vi "fetch_position_feedback.vi"(8 "error in (no error)":errorcluster, 11 "ScanHeadDL090202 in":refnum<class "ScanHeadDL090202.lvclass">) -> (0 "error out":errorcluster, 3 "ScanHeadDL090202 out":refnum<class "ScanHeadDL090202.lvclass">)   [LabVIEW 2010, in "ScanHeadDL090202.lvclass"]
uses:
  ScanHeadDL090202.lvclass
  common/enumerations/functional_global_action_enum.ctl
  Trajectory/TrajectoryDL091126GenericVoxel/TrajectoryDL091126GenericVoxel/TrajectoryDL091126GenericVoxel.lvclass
  common/classes/ErrorController/ErrorController/ErrorController.lvclass
  internal_trigger_enum.ctl
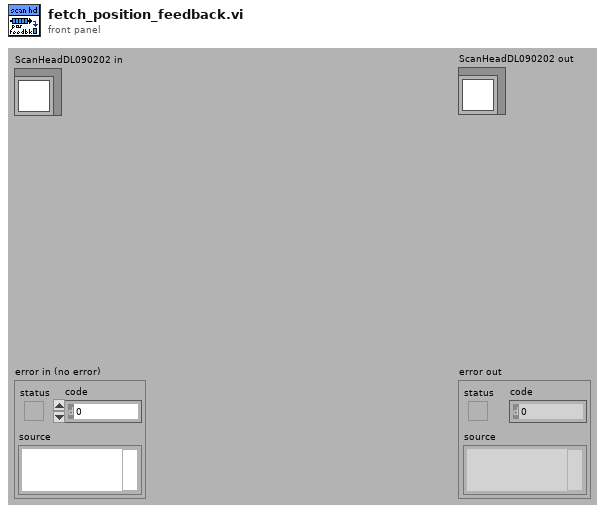
[diagram p1: front panel]
types:
  T1 = typedef "functional_global_action_enum.ctl" = enum16{"get", "set", "reset"}
  T2 = typedef "ScanHeadDL090202.lvclass/internal_trigger_enum.ctl" = enum16{"NULL", "initialise", "terminate", "start scanning", "stop scanning", "scale", "rotate", "tilt", "translate", "update modifiers", "fetch trajectory", "set run mode", "initialise scanners", "terminate scanners", "generate trajectory", "prepare writing", "write", "calculate scanner delays", "fetch position feedback"}
  T3 = typedef "pixel_raw_data_array.ctl" = dbl[][]
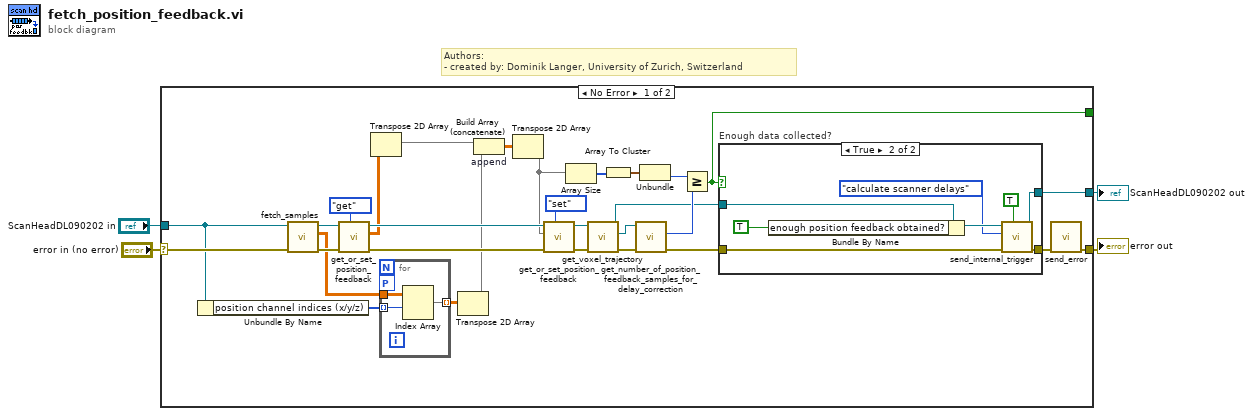
[diagram p0: block diagram]
diagram:
  # "Authors: \n- created by: Dominik Langer, University of Zurich, Switzerland"
  n1 = case shown="No Error" "error in (no error)" {
    selector: "error in (no error)" -> [w9 w49]
    tunnel: [w11 w49] -> w3
    tunnel: [w30 w48] -> w1
    tunnel: "ScanHeadDL090202 in" -> [w8 w48]
    tunnel: [w27 _] -> _
    frame No Error {
      n2 = Unbundle By Name(w8) -> ("position channel indices (x/y/z)"=w25:i32[])
      n3 = call-dynamic "fetch_samples.vi"("error in (no error)"=w9, "GenericToplevelComponent in"=w8) -> ("error out"=w7:errorcluster, "channels raw data block"=w5:T3, "GenericToplevelComponent out"=w6:refnum<class "ScanHeadDL090202.lvclass">)  [unwired: 6 in, 1 out]
      n4 = call-dynamic "get_or_set_position_feedback.vi"("action"=functional_global_action_enum."get", "error in (no error)"=w7, "ScanHeadDL090202 in"=w6) -> ("error out"=w34:errorcluster, "position feedback data out"=w17:T3, "ScanHeadDL090202 out"=w33:refnum<class "ScanHeadDL090202.lvclass">)  [unwired: 6 in]
      n5 = Transpose 2D Array(2D array=w17) -> (transposed array=w16:T3)
      n6 = for {
        tunnel: w25 -> [w36] mode=indexing
        tunnel: w5 -> [w37]
        workers-P: _ -> [_]
        tunnel: [w35] -> w13 mode=indexing
        n7 = Index Array(array=w37, index (row)=w36) -> (element=w35:dbl[])  [unwired: 1 in]
      }
      n8 = Transpose 2D Array(2D array=w13) -> (transposed array=w14:dbl[][])
      n9 = Build Array (concatenate) "append"(w16, w14) -> (w15:T3)
      n10 = Transpose 2D Array(2D array=w15) -> (transposed array=w12:T3)
      n11 = call-dynamic "get_or_set_position_feedback.vi"("action"=functional_global_action_enum."set", "error in (no error)"=w34, "position feedback data in"=w12, "ScanHeadDL090202 in"=w33) -> ("error out"=w24:errorcluster, "ScanHeadDL090202 out"=w20:refnum<class "ScanHeadDL090202.lvclass">)  [unwired: 5 in, 1 out]
      n12 = Array Size(array=w12) -> (size(s)=w29:i32[])
      n13 = call-dynamic "get_voxel_trajectory.vi"("error in (no error)"=w24, "ScanHeadDL090202 in"=w20) -> ("error out"=w22:errorcluster, "trajectory"=w21:refnum<class "TrajectoryDL091126GenericVoxel.lvclass">, "ScanHeadDL090202 out"=w18:refnum<class "ScanHeadDL090202.lvclass">)  [unwired: 7 in]
      n14 = Array To Cluster(array=w29) -> (cluster=w28:cluster{"[0]":i32, "[1]":i32})
      n15 = call-dynamic "get_number_of_position_feedback_samples_for_delay_correction.vi"("error in (no error)"=w22, "TrajectoryDL091126GenericVoxel in"=w21) -> ("error out"=w23:errorcluster, "number of pixels required"=w19:i32)  [unwired: 7 in, 1 out]
      n16 = Unbundle(w28) -> ("[1]"=w26:i32)  [unwired: 1 out]
      n17 = Greater Or Equal?(x=w26, y=w19) -> (x >= y?=w27:bool)
      n18 = case "Enough data collected?" shown="True" w27 {
        tunnel: w23 -> [w38 w44]
        tunnel: [w38 w43] -> w10
        tunnel: w18 -> [w39 w47]
        tunnel: [w39 w41] -> w30
        frame False {
        }
        frame True {
          n19 = Bundle By Name(cluster=w47, "enough position feedback obtained?"=TRUE ("scanner delays calculated?")) -> (w42:refnum<class "ScanHeadDL090202.lvclass">)
          n20 = call-dynamic "send_internal_trigger.vi"("ensure unique insertion?"=TRUE, "error in (no error)"=w44, "trigger"=internal_trigger_enum."calculate scanner delays", "DL090202ScanHead in"=w42) -> ("error out"=w43:errorcluster, "DL090202ScanHead out"=w41:refnum<class "ScanHeadDL090202.lvclass">)  [unwired: 4 in, 2 out]
        }
      }
      n21 = call "send_error.vi"("error in (no error)"=w10) -> ("error out"=w11:errorcluster)  [unwired: 10 in]
    }
    frame Error {
    }
  }
  "error out" <- w3
  "ScanHeadDL090202 out" <- w1
